vi "Force_3_1.vi"() -> ()   [LabVIEW 2020]
uses:
  Support/Controls/Cmd_Mouse Popup.ctl
  Support/Controls/Clst_Initialize Input.ctl
  Support/Controls/Cmd_Var Data IO.ctl
  Variables/Global_Cal Info.vi
panel:
  in  "Measured_ADJ":string[][](table) caption="● 푸쉬풀 게이지 지시값 (조정후)"
  out "구분":string
  out "분해능":string
  out "std set":string[][](table) caption="○ 분동 세트"
  out "표시방식":string
  in  "Spec 변경":bool
  in  "Random":bool
  out "Spec":string[][](table)
  out "제목":string
  out "에러 출력":errorcluster
  out "Condition":string[][](table) caption="○ 상대지시 오차 교정"
  in  "최소눈금":string(combo)
  out "단위":string
  out "최대용량":string
  in  "Measured":string[][](table) caption="● 푸쉬풀 게이지 지시값"
  out "Load?":bool
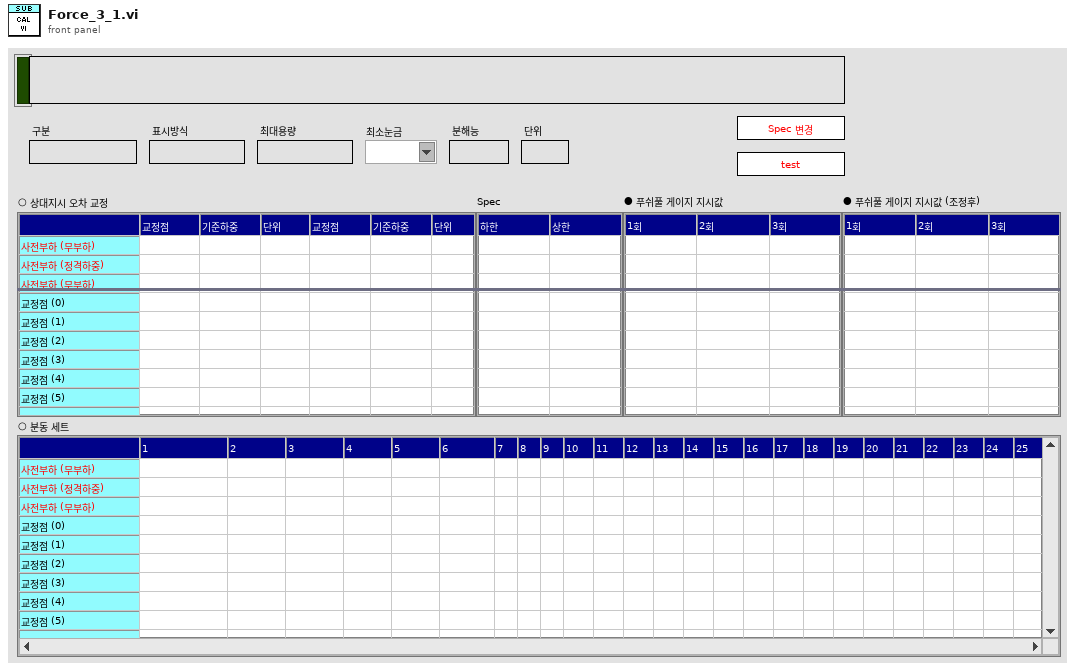
[diagram p1: front panel]
types:
  T1 = typedef "Cmd_Mouse Popup.ctl" = enum16{"활성화", "메뉴선택"}
  T2 = cluster{"Shift":bool, "Ctrl":bool, "Alt":bool, "Cmd":bool, "Opt":bool}
  T3 = typedef "Clst_Initialize Input.ctl" = cluster{"Initialize 1":cluster{"Condition":refnum<vi>[], "Spec":refnum<vi>[], "Measured":refnum<vi>[], "Resolution":refnum<vi>[], "Func_ext":string, "제목":refnum<vi>, "Measured_ADJ":refnum<vi>[]}, "Initialize 2":cluster{"문자열":refnum<vi>[], "콤보박스":refnum<vi>[], "링":refnum<vi>[], "열거형":refnum<vi>[], "테이블":refnum<vi>[], "여러열":refnum<vi>[], "디지털(DBL)":refnum<vi>[], "3D string":refnum<vi>[], "ctrl":refnum<vi>[], "boolean":refnum<vi>[]}}
  T4 = typedef "Cmd_Var Data IO.ctl" = enum16{"Condition", "Condition Default", "Condition_Temp", "Resolution", "Resolution Default", "Resolution Old", "Spec", "Spec Default", "Spec Old", "Spec Temp", "Result", "Result2", "Result3", "Result_Temp", "Result_ADJ", "Result_ADJ2", "STD1", "STD2", "STD3", "STD4", "STD5", "STD Temp", "CMC", "CMC Default"}
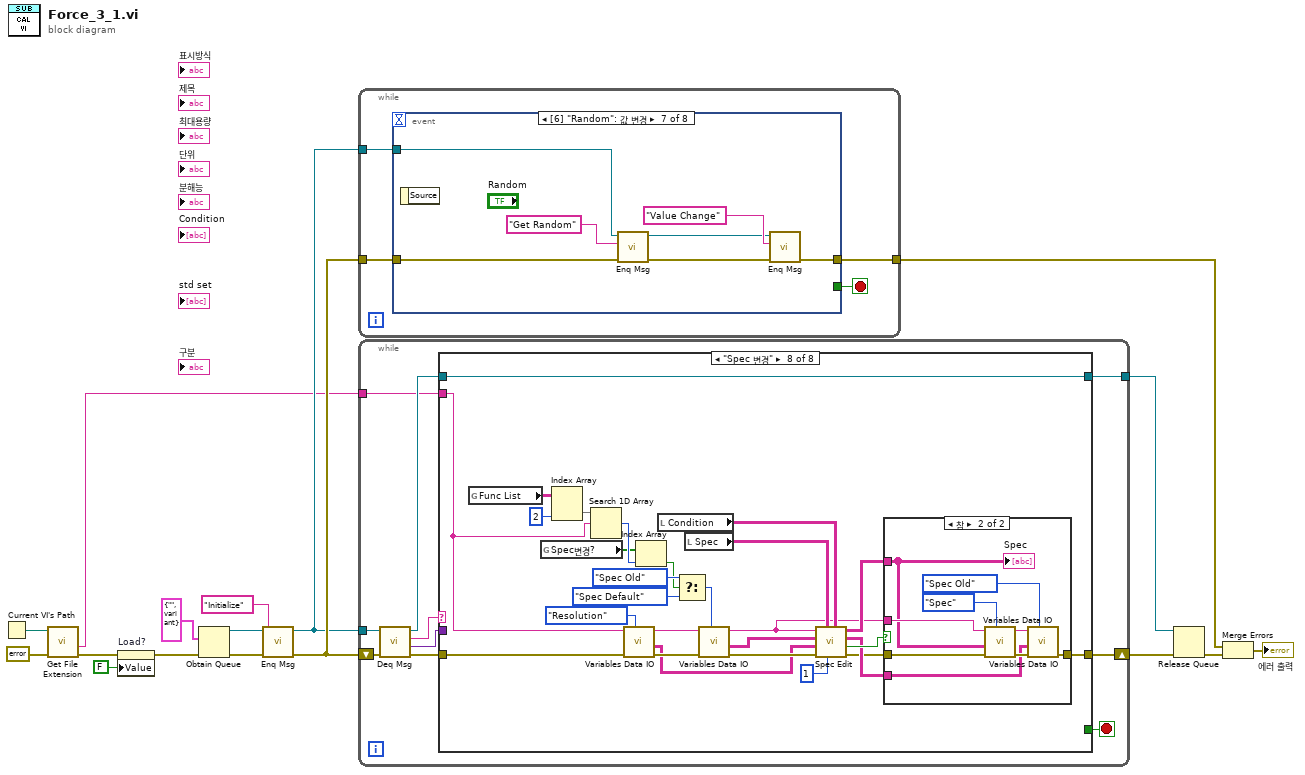
[diagram p0: block diagram]
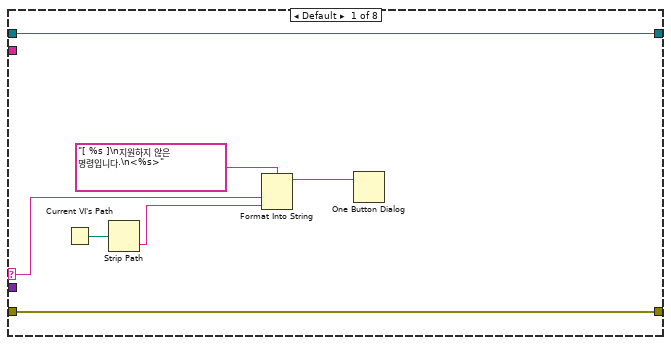
[diagram p2: hidden frame]
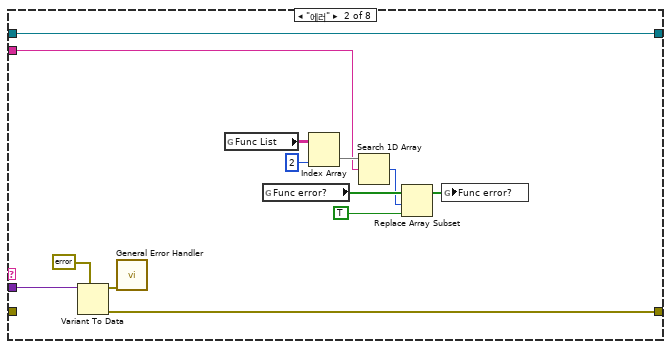
[diagram p3: hidden frame]
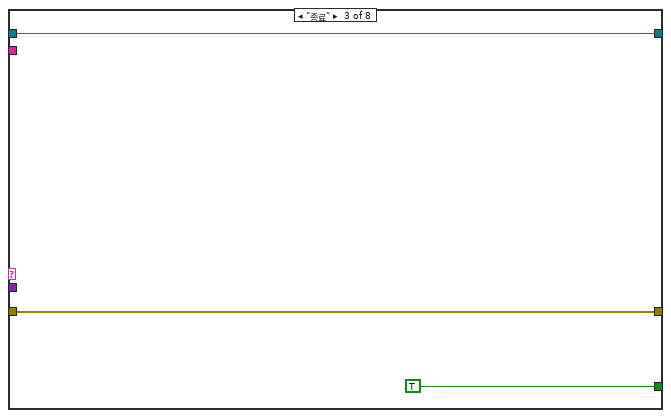
[diagram p4: hidden frame]
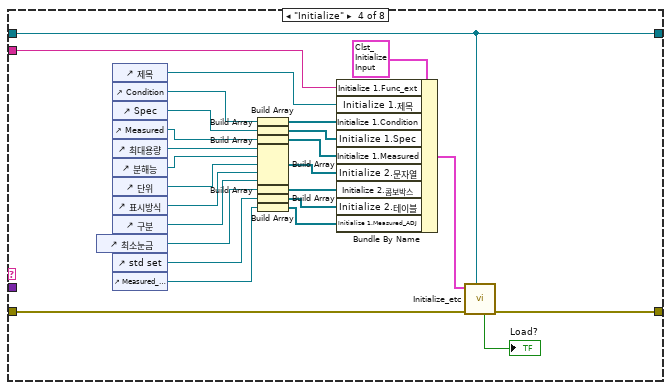
[diagram p5: hidden frame]
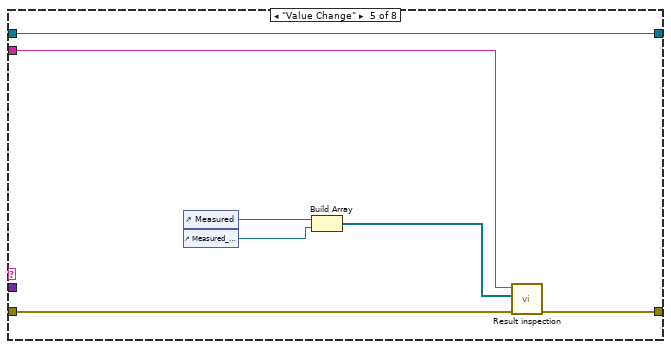
[diagram p6: hidden frame]
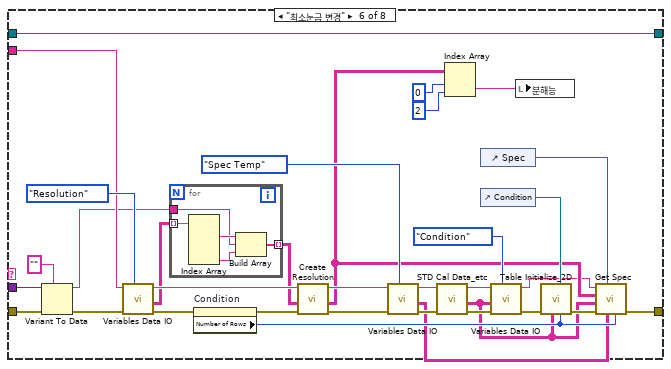
[diagram p7: hidden frame]
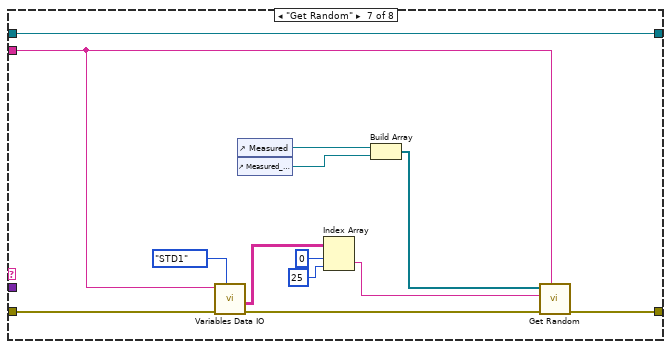
[diagram p8: hidden frame]
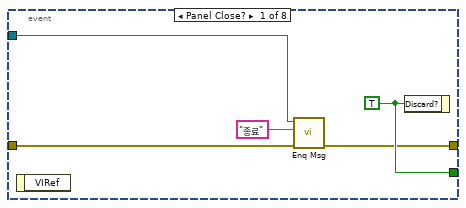
[diagram p10: hidden frame]
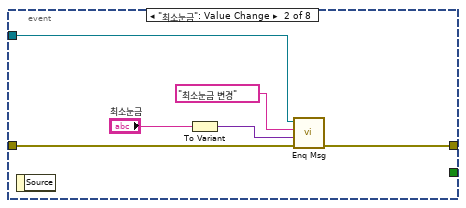
[diagram p11: hidden frame]
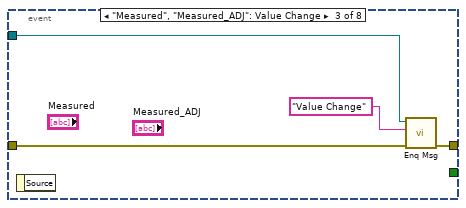
[diagram p12: hidden frame]
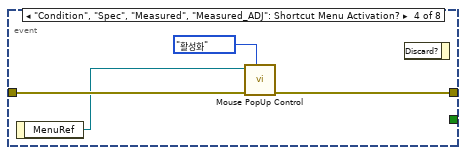
[diagram p13: hidden frame]
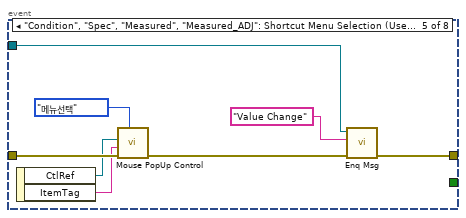
[diagram p14: hidden frame]
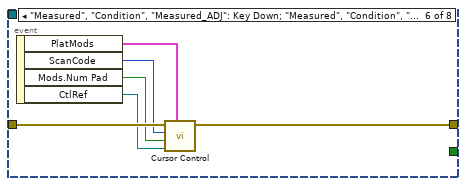
[diagram p15: hidden frame]
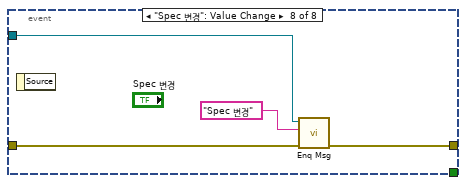
[diagram p16: hidden frame]
diagram:
  n1 = Current VI's Path() -> (path=w5:path)
  n2 = call <vilib>:"Get File Extension.vi"("error in (no error)"=errorcluster {"status"=FALSE, "code"=0, "source"=""} ("에러 상수"), "file"=w5) -> ("error out"=w3:errorcluster, "filename without extension"=w4:string)  [unwired: 5 in, 3 out]
  n3 = property on="Load?" class="Bool (엄격한)"(error in=w3, "Value"=FALSE ("Load?")) -> (error out=w2:errorcluster)  [unwired: 1 in, 1 out]
  n4 = Obtain Queue(element data type=cluster{"메세지":string, "값":variant} {"메세지"="", "값"=variant} ("Message Cluster"), error in (no error)=w2) -> (queue out=w14:refnum<queue>, error out=w16:errorcluster)  [unwired: 3 in, 1 out]
  n5 = call "Enq Msg.vi"("에러 입력(에러 없음)"=w16, "메세지"="Initialize", "큐 입력"=w14) -> ("에러 출력"=w15:errorcluster, "큐 출력"=w12:refnum<queue>)  [unwired: 7 in]
  n6 = while {
    tunnel: w15 -> [w19]
    tunnel: w12 -> [w20]
    tunnel: [w18] -> w9
    stop <- w21 stop-if-true
    n7 = event shown="[6] \"Random\": 값 변경" {
      selector: _ -> [_ _ _ _ _ _ _ _]
      dyn-events: _ -> [_ _ _ _ _ _ _ _]
      timeout: _ -> [_ _ _ _ _ _ _ _]
      tunnel: [w26 _ _ _ _ _ _ _] -> w21
      tunnel: w20 -> [w24 w31 w35 _ w42 _ w56 w62]
      tunnel: w19 -> [w25 w32 w36 w39 w47 w54 w57 w64]
      tunnel: [w22 w29 w33 w38 w41 w53 w55 w63] -> w18
      event Panel Close? {
        w26 = TRUE ("버림?")
        n8 = event-data() -> ()  [unwired: 1 in, 1 out]
        n9 = call "Enq Msg.vi"("에러 입력(에러 없음)"=w25, "메세지"="종료", "큐 입력"=w24) -> ("에러 출력"=w22:errorcluster)  [unwired: 7 in, 1 out]
        n10 = event-data("Discard?"=w26) -> ()  [unwired: 1 in, 1 out]
      }
      event "최소눈금": Value Change {
        n11 = event-data() -> ()  [unwired: 1 in, 1 out]
        n12 = To Variant(anything="최소눈금") -> (Variant=w27:variant)
        n13 = call "Enq Msg.vi"("에러 입력(에러 없음)"=w32, "값"=w27, "메세지"="최소눈금 변경", "큐 입력"=w31) -> ("에러 출력"=w29:errorcluster)  [unwired: 6 in, 1 out]
      }
      event "Measured", "Measured_ADJ": Value Change {
        n14 = event-data() -> ()  [unwired: 1 in, 1 out]
        n15 = call "Enq Msg.vi"("에러 입력(에러 없음)"=w36, "메세지"="Value Change", "큐 입력"=w35) -> ("에러 출력"=w33:errorcluster)  [unwired: 7 in, 1 out]
      }
      event "Condition", "Spec", "Measured", "Measured_ADJ": Shortcut Menu Activation? {
        n16 = event-data() -> ("MenuRef"=w37:refnum<k9>)  [unwired: 1 in]
        n17 = call "Mouse PopUp Control.vi"("type"=Cmd_Mouse_Popup."활성화", "error in"=w39, "메뉴 참조"=w37) -> ("error out"=w38:errorcluster)  [unwired: 8 in]
        n18 = event-data() -> ()  [unwired: 2 in, 1 out]
      }
      event "Condition", "Spec", "Measured", "Measured_ADJ": Shortcut Menu Selection (User) {
        n19 = event-data() -> ("CtlRef"=w45:refnum<vi>, "ItemTag"=w46:string)  [unwired: 1 in]
        n20 = call "Mouse PopUp Control.vi"("type"=Cmd_Mouse_Popup."메뉴선택", "error in"=w47, "아이템 태그"=w46, "Tbl 참조 번호"=w45) -> ("error out"=w43:errorcluster)  [unwired: 7 in]
        n21 = call "Enq Msg.vi"("에러 입력(에러 없음)"=w43, "메세지"="Value Change", "큐 입력"=w42) -> ("에러 출력"=w41:errorcluster)  [unwired: 7 in, 1 out]
      }
      event "Measured", "Condition", "Measured_ADJ": Key Down; "Measured", "Condition", "Measured_ADJ": Key Repeat {
        n22 = event-data() -> ("PlatMods"=w49:T2, "ScanCode"=w52:i16, "Mods.Num Pad"=w51:bool, "CtlRef"=w50:refnum<vi>)  [unwired: 1 in]
        n23 = call "Cursor Control.vi"("플랫폼 조합키"=w49, "참조"=w50, "Num Pad"=w51, "ScanCode"=w52, "error in"=w54) -> ("error out"=w53:errorcluster)  [unwired: 5 in, 1 out]
      }
      event "Random": Value Change {
        n24 = event-data() -> ()  [unwired: 1 in, 1 out]
        n25 = call "Enq Msg.vi"("에러 입력(에러 없음)"=w57, "메세지"="Get Random", "큐 입력"=w56) -> ("에러 출력"=w59:errorcluster, "큐 출력"=w60:refnum<queue>)  [unwired: 7 in]
        n26 = call "Enq Msg.vi"("에러 입력(에러 없음)"=w59, "메세지"="Value Change", "큐 입력"=w60) -> ("에러 출력"=w55:errorcluster)  [unwired: 7 in, 1 out]
      }
      event "Spec 변경": Value Change {
        n27 = event-data() -> ()  [unwired: 1 in, 1 out]
        n28 = call "Enq Msg.vi"("에러 입력(에러 없음)"=w64, "메세지"="Spec 변경", "큐 입력"=w62) -> ("에러 출력"=w63:errorcluster)  [unwired: 7 in, 1 out]
      }
    }
  }
  n29 = while {
    shift-right: [w75] -> w11
    shift-left: w15 -> [w74]
    tunnel: w12 -> [w72]
    tunnel: [w67] -> w10
    tunnel: w4 -> [w66]
    stop <- w68 stop-if-true
    n30 = call "Deq Msg.vi"("에러 입력(에러 없음)"=w74, "큐 입력"=w72) -> ("에러 출력"=w73:errorcluster, "값"=w69:variant, "메세지"=w71:string, "큐 출력"=w70:refnum<queue>)  [unwired: 6 in]
    n31 = case shown="\"Spec 변경\"" w71 {
      selector: w71 -> [w78 _ _ _ _ _ _ _]
      tunnel: w73 -> [w82 _ w98 w110 w126 w164 w178 w187]
      tunnel: [w82 w92 w98 w107 w130 w149 w181 w188] -> w75
      tunnel: w70 -> [w81 w91 w96 w112 w131 w165 w183 w210]
      tunnel: w69 -> [_ w93 _ _ _ w163 _ _]
      tunnel: [_ _ TRUE ("버림?") _ _ _ _ _] -> w68
      tunnel: [w81 w91 w96 w112 w131 w165 w183 w210] -> w67
      tunnel: w66 -> [_ w83 _ w106 w129 w159 w179 w186]
      frame Default {
        n32 = Current VI's Path() -> (path=w77:path)
        n33 = Strip Path(path=w77) -> (name=w76:string)  [unwired: 1 out]
        n34 = Format Into String(format string="[ %s ]\n지원하지 않은 명령입니다.\n<%s>" ("메시지"), w78, w76) -> (resulting string=w79:string)  [unwired: 2 in, 1 out]
        n35 = One Button Dialog(message=w79) -> ()  [unwired: 1 in, 1 out]
      }
      frame "에러" {
        n36 = Variant To Data(type=errorcluster {"status"=FALSE, "code"=0, "source"=""} ("에러 출력"), Variant=w93) -> (data=w95:errorcluster, error out=w92:errorcluster)  [unwired: 1 in]
        n37 = call <vilib>:"General Error Handler.vi"("error in (no error)"=w95) -> ()  [unwired: 10 in, 5 out]
        n38 = global read "Global_Cal Info.vi" "Func List"() -> (w89:string[][])
        n39 = global read "Global_Cal Info.vi" "Func error?"() -> (w86:bool[])
        n40 = Index Array(array=w89, index (col)=2 ("비활성화된 인덱스 (열)")) -> (element=w88:string[])  [unwired: 1 in]
        n41 = Search 1D Array(1D array=w88, element=w83) -> (index of element=w85:i32)  [unwired: 1 in]
        n42 = Replace Array Subset(array=w86, new element=TRUE ("새 원소/부분배열"), index=w85) -> (w84:bool[])
        n43 = global write "Global_Cal Info.vi" "Func error?"(w84) -> ()
      }
      frame "종료" {
      }
      frame "Initialize" {
        n44 = control-ref of="최소눈금"() -> (w118:refnum<vi>)
        n45 = control-ref of="제목"() -> (w116:refnum<vi>)
        n46 = control-ref of="Condition"() -> (w111:refnum<vi>)
        n47 = control-ref of="Spec"() -> (w109:refnum<vi>)
        n48 = control-ref of="Measured"() -> (w120:refnum<vi>)
        n49 = control-ref of="최대용량"() -> (w115:refnum<vi>)
        n50 = control-ref of="분해능"() -> (w103:refnum<vi>)
        n51 = control-ref of="단위"() -> (w114:refnum<vi>)
        n52 = control-ref of="표시방식"() -> (w108:refnum<vi>)
        n53 = control-ref of="구분"() -> (w102:refnum<vi>)
        n54 = control-ref of="std set"() -> (w104:refnum<vi>)
        n55 = control-ref of="Measured_ADJ"() -> (w101:refnum<vi>)
        n56 = Build Array(w111) -> (w122:refnum<vi>[])
        n57 = Build Array(w109) -> (w113:refnum<vi>[])
        n58 = Build Array(w120) -> (w121:refnum<vi>[])
        n59 = Build Array(w115, w103, w114, w108, w102) -> (w119:refnum<vi>[])
        n60 = Build Array(w118) -> (w117:refnum<vi>[])
        n61 = Build Array(w104) -> (w105:refnum<vi>[])
        n62 = Build Array(w101) -> (w100:refnum<vi>[])
        n63 = Bundle By Name(cluster=T3 {"Initialize 1"={"Condition"=[], "Spec"=[], "Measured"=[], "Resolution"=[], "Func_ext"="", "제목"=refnum, "Measured_ADJ"=[]}, "Initialize 2"={"문자열"=[], "콤보박스"=[], "링"=[], "열거형"=[], "테이블"=[], "여러열"=[], "디지털(DBL)"=[], "3D string"=[], "ctrl"=[], "boolean"=[]}} ("입력 클러스터"), "Initialize 1.Func_ext"=w106, "Initialize 1.제목"=w116, "Initialize 1.Condition"=w122, "Initialize 1.Spec"=w113, "Initialize 1.Measured"=w121, "Initialize 2.문자열"=w119, "Initialize 2.콤보박스"=w117, "Initialize 2.테이블"=w105, "Initialize 1.Measured_ADJ"=w100) -> (w123:T3)
        n64 = call "Initialize_etc.vi"("큐 입력"=w112, "error in"=w110, "입력 클러스터"=w123) -> ("error out"=w107:errorcluster, "Load?"=→"Load?":bool)  [unwired: 6 in, 1 out]
      }
      frame "Value Change" {
        n65 = control-ref of="Measured"() -> (w128:refnum<vi>)
        n66 = control-ref of="Measured_ADJ"() -> (w125:refnum<vi>)
        n67 = Build Array(w128, w125) -> (w127:refnum<vi>[])
        n68 = call "Result inspection.vi"("error in"=w126, "Ref. Data (Inspection)"=w127, "Func ext"=w129) -> ("error out"=w130:errorcluster)  [unwired: 5 in, 3 out]
      }
      frame "최소눈금 변경" {
        n69 = Variant To Data(error in=w164, type="", Variant=w163) -> (data=w157:string, error out=w158:errorcluster)
        n70 = call "Variables Data IO.vi"("Select"=Cmd_Var_Data_IO."Resolution", "error in"=w158, "Func_ext"=w159) -> ("error out"=w142:errorcluster, "Data Out"=w156:string[][], "Func_ext Out"=w160:string)  [unwired: 6 in]
        n71 = for {
          tunnel: w156 -> [w170] mode=indexing
          tunnel: w157 -> [w168]
          tunnel: [w166] -> w155 mode=indexing
          n72 = Index Array(array=w170) -> (element #1=w169:string, element #4=w167:string)  [unwired: 4 in, 2 out]
          n73 = Build Array(w169, w168, w167) -> (w166:string[])
        }
        n74 = property on="Condition" class="Tbl (엄격한)"(error in=w142) -> (error out=w141:errorcluster, "Number of Rows"=w136:u32)  [unwired: 1 in, 1 out]
        n75 = call "Create Resolution.vi"("에러 입력(에러 없음)"=w141, "Resolution"=w155, "Func_ext"=w160) -> ("에러 출력"=w146:errorcluster, "Resolution Out"=w133:string[][], "Func_ext 출력"=w145:string)  [unwired: 6 in]
        n76 = call "Variables Data IO.vi"("Select"=Cmd_Var_Data_IO."Spec Temp", "error in"=w146, "Func_ext"=w145) -> ("error out"=w144:errorcluster, "Data Out"=w135:string[][], "Func_ext Out"=w143:string)  [unwired: 6 in]
        n77 = call "STD Cal Data_etc.vi"("error in"=w144, "Func_ext"=w143) -> ("error out"=w152:errorcluster, "Data Out"=w134:string[][], "Func_ext Out"=w153:string)  [unwired: 5 in, 2 out]
        n78 = Index Array(array=w133, index (row)=0 ("인덱스 (행)"), index (col)=2 ("비활성화된 인덱스 (열)")) -> (element=w138:string)
        n79 = control-ref of="Spec"() -> (w148:refnum<vi>)
        n80 = control-ref of="Condition"() -> (w137:refnum<vi>)
        n81 = call "Variables Data IO.vi"("Select"=Cmd_Var_Data_IO."Condition", "error in"=w152, "Data In"=w134, "Func_ext"=w153) -> ("error out"=w151:errorcluster, "Func_ext Out"=w132:string)  [unwired: 5 in, 1 out]
        n82 = local write "분해능"(w138) -> ()
        n83 = call "Table Initialize_2D.vi"("행의 개수"=w136, "Table Ref"=w137, "Value"=w134, "에러 입력"=w151) -> ("에러 출력"=w154:errorcluster)  [unwired: 5 in, 2 out]
        n84 = call "Get Spec.vi"("NumRows"=w136, "Spec in"=w135, "Spec Ref."=w148, "error in"=w154, "Condition in"=w134, "Resolution in"=w133, "Func_ext"=w132) -> ("error out"=w149:errorcluster)  [unwired: 4 out]
      }
      frame "Get Random" {
        n85 = call "Variables Data IO.vi"("Select"=Cmd_Var_Data_IO."STD1", "error in"=w178, "Func_ext"=w179) -> ("error out"=w177:errorcluster, "Data Out"=w175:string[][])  [unwired: 6 in, 1 out]
        n86 = control-ref of="Measured"() -> (w180:refnum<vi>)
        n87 = control-ref of="Measured_ADJ"() -> (w171:refnum<vi>)
        n88 = Index Array(array=w175, index (row)=0 ("인덱스 (행)"), index (col)=25 ("비활성화된 인덱스 (열)")) -> (element=w172:string)
        n89 = Build Array(w180, w171) -> (w182:refnum<vi>[])
        n90 = call "Get Random.vi"("Func_Ext"=w179, "에러 입력"=w177, "분해능"=w172, "Meas"=w182) -> ("에러 출력"=w181:errorcluster)  [unwired: 6 in, 1 out]
      }
      frame "Spec 변경" {
        n91 = global read "Global_Cal Info.vi" "Func List"() -> (w194:string[][])
        n92 = global read "Global_Cal Info.vi" "Spec변경?"() -> (w190:bool[])
        n93 = Index Array(array=w194, index (col)=2 ("비활성화된 인덱스 (열)")) -> (element=w192:string[])  [unwired: 1 in]
        n94 = Search 1D Array(1D array=w192, element=w186) -> (index of element=w191:i32)  [unwired: 1 in]
        n95 = call "Variables Data IO.vi"("Select"=Cmd_Var_Data_IO."Resolution", "error in"=w187, "Func_ext"=w186) -> ("error out"=w201:errorcluster, "Data Out"=w184:string[][], "Func_ext Out"=w200:string)  [unwired: 6 in]
        n96 = Index Array(array=w190, index=w191) -> (element=w195:bool)
        n97 = local read "Condition"() -> (w204:string[][])
        n98 = Select(t=Cmd_Var_Data_IO."Spec Old" ("Select"), s=w195, f=Cmd_Var_Data_IO."Spec Default" ("Select")) -> (s? t:f=w189:T4)
        n99 = local read "Spec"() -> (w205:string[][])
        n100 = call "Variables Data IO.vi"("Select"=w189, "error in"=w201, "Func_ext"=w200) -> ("error out"=w199:errorcluster, "Data Out"=w185:string[][], "Func_ext Out"=w202:string)  [unwired: 6 in]
        n101 = call "Spec Edit.vi"("Condition"=w204, "열번호(기준값)"=1 ("기준열(0)"), "Spec Value"=w205, "에러 입력(에러 없음)"=w199, "Resolution"=w184, "Spec Default"=w185, "Func_ext"=w202) -> ("에러 출력"=w203:errorcluster, "변경?"=w209:bool, "Spec Default out"=w208:string[][], "Spec 출력"=w206:string[][])  [unwired: 1 in]
        n102 = case shown="참" w209 {
          tunnel: w203 -> [w211 w219]
          tunnel: [w211 w216] -> w188
          tunnel: w206 -> [_ w212]
          tunnel: w202 -> [_ w218]
          tunnel: w208 -> [_ w213]
          frame False {
          }
          frame True {
            n103 = call "Variables Data IO.vi"("Select"=Cmd_Var_Data_IO."Spec", "error in"=w219, "Data In"=w212, "Func_ext"=w218) -> ("error out"=w217:errorcluster, "Func_ext Out"=w214:string)  [unwired: 5 in, 1 out]
            n104 = call "Variables Data IO.vi"("Select"=Cmd_Var_Data_IO."Spec Old", "error in"=w217, "Data In"=w213, "Func_ext"=w214) -> ("error out"=w216:errorcluster)  [unwired: 5 in, 2 out]
            "Spec" <- w212
          }
        }
      }
    }
  }
  n105 = Release Queue(queue=w10, error in (no error)=w11) -> (error out=w8:errorcluster)  [unwired: 1 in, 2 out]
  n106 = Merge Errors(w9, w8) -> (→"에러 출력":errorcluster)
